vi "addDeleteRowsColour.vi"(8 "error in (no error)":errorcluster, 9 "Add?":bool, 10 "index":i32, 11 "reference in":refnum<class "Project Panels.lvclass">) -> (0 "error out":errorcluster, 3 "reference out":refnum<class "Project Panels.lvclass">)   [LabVIEW 2016, in "Project Panels.lvclass"]
uses:
  Project Panels.lvclass
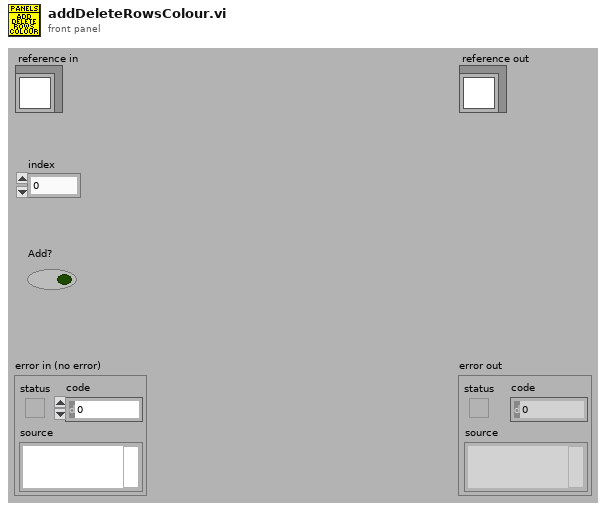
[diagram p1: front panel]
types:
  T1 = typedef "Project Panels.lvclass/ObjectAttributesRef.ctl" = refnum<data-value>
  T2 = typedef "Project Panels.lvclass/ObjectAttributes.ctl" = cluster{"MyAttribute":dbl, "device_controller_ref":refnum<class "Devices Controller.lvclass">, "file_controller_ref":refnum<class "File Controller.lvclass">, "item_controller_ref":refnum<class "Items Controller.lvclass">, "item_tables":cluster{"checkIN":string[][], "checkOUT":string[][], "storage":string[][]}, "quickbook_table":cluster{"notes":string[][]}, "notification_controller_ref":refnum<class "Notification Controller.lvclass">, "partstracking_controller_ref":refnum<class "PartsTracking Controller.lvclass">, "product_tables":cluster{"k4b2":string[][], "fitmate":string[][], "RMR":string[][], "CPET":string[][], "BP":string[][], "PP":string[][], "k5":string[][], "bb-pft":string[][]}, "rowsColour":u32[], "low_resolution?":bool, "run_python?":bool}
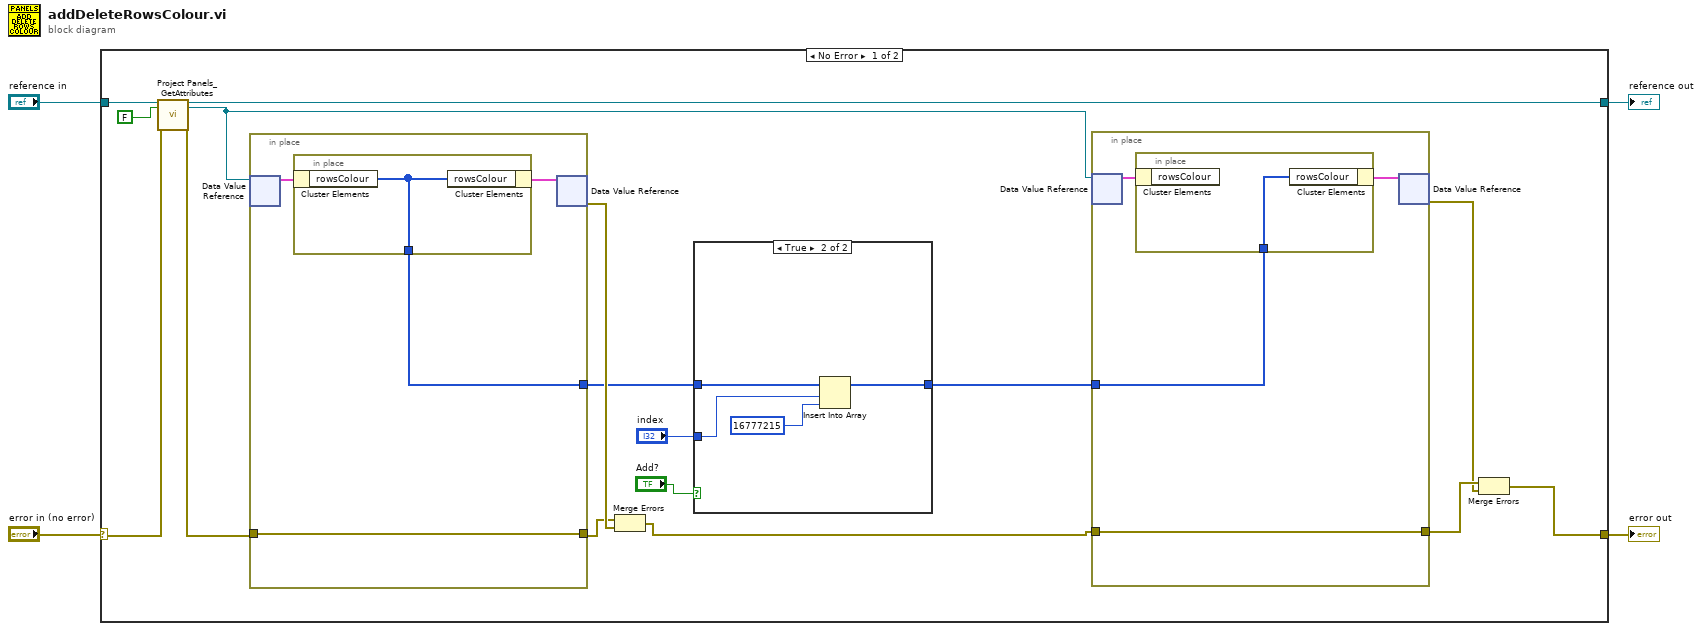
[diagram p0: block diagram]
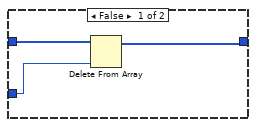
[diagram p2: hidden frame]
diagram:
  n1 = case shown="No Error" "error in (no error)" {
    selector: "error in (no error)" -> [w16 w39]
    tunnel: [w6 w39] -> w3
    tunnel: [w14 w38] -> w1
    tunnel: "reference in" -> [w18 w38]
    frame No Error {
      n2 = call "Project Panels_GetAttributes.vi"("reference in"=w18, "return data? (T)"=FALSE, "error in (no error)"=w16) -> ("reference out"=w14:refnum<class "Project Panels.lvclass">, "attributes ref"=w8:T1, "error out"=w15:errorcluster)  [unwired: 13 in, 1 out]
      n3 = in-place {
        in-place-border: w15 -> [w34]
        in-place-border: [w34] -> w19
        in-place-border: [w33] -> w11
        n4 = in-place-dvr #1(w8) -> (w35:T2)  [unwired: 1 out]
        n5 = in-place {
          in-place-border: [w37] -> w33
          n6 = in-place-cluster #2(w35) -> ("rowsColour"=w37:u32[])
          n7 = in-place-cluster #2("rowsColour"=w37) -> (w36:T2)
        }
        n8 = in-place-dvr #1(w36) -> (w20:errorcluster)  [unwired: 1 out]
      }
      n9 = Merge Errors(w19, w20) -> (w7:errorcluster)
      n10 = case shown="True" "Add?" {
        tunnel: "index" -> [w26 w31]
        tunnel: w11 -> [w28 w32]
        tunnel: [w27 w29] -> w5
        frame False {
          n11 = Delete From Array(array=w28, index=w26) -> (array with subset deleted=w27:u32[])  [unwired: 1 in, 1 out]
        }
        frame True {
          n12 = Insert Into Array(array=w32, index=w31, new element=u32 16777215 ("new element/subarray")) -> (w29:u32[])
        }
      }
      n13 = in-place {
        in-place-border: w7 -> [w22]
        in-place-border: [w22] -> w10
        in-place-border: w5 -> [w21]
        n14 = in-place-dvr #3(w8) -> (w23:T2)  [unwired: 1 out]
        n15 = in-place {
          in-place-border: w21 -> [w25]
          n16 = in-place-cluster #4(w23) -> ()  [unwired: 1 out]
          n17 = in-place-cluster #4("rowsColour"=w25) -> (w24:T2)
        }
        n18 = in-place-dvr #3(w24) -> (w9:errorcluster)  [unwired: 1 out]
      }
      n19 = Merge Errors(w10, w9) -> (w6:errorcluster)
    }
    frame Error {
    }
  }
  "error out" <- w3
  "reference out" <- w1
